vi "Encoders Per Iteration Calculator 2.vi"(6 "encoder":dbl, 8 "iteration in":dbl, 9 "total iterations":dbl, 10 "speed in":dbl, 11 "on in":bool) -> (0 "iteration out":dbl, 1 "encoders per iteration":dbl, 2 "speed out":dbl, 3 "on out":bool)   [LabVIEW 2014]
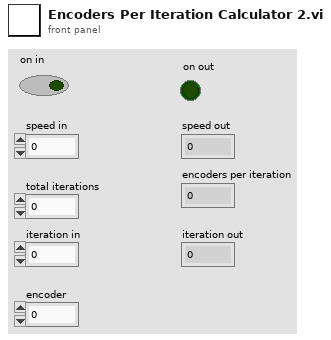
[diagram p1: front panel]
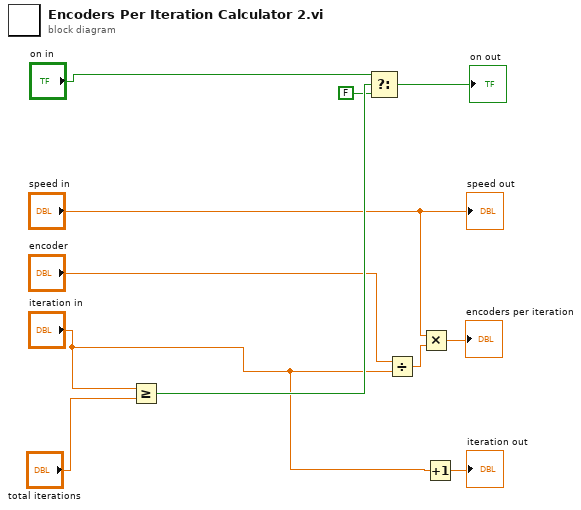
[diagram p0: block diagram]
diagram:
  n1 = Greater Or Equal?(x="iteration in", y="total iterations") -> (x >= y?=w9:bool)
  n2 = Select(t="on in", s=w9, f=FALSE) -> (s? t:f=→"on out":bool)
  n3 = Divide(x="encoder", y="iteration in") -> (x/y=w6:dbl)
  n4 = Multiply(x="speed in", y=w6) -> (x*y=→"encoders per iteration":dbl)
  n5 = Increment(x="iteration in") -> (x+1=→"iteration out":dbl)
  "speed out" <- "speed in"
